vi "RandomizeTargetSequence.vi"(10 "NumRepetitions":i32, 11 "Inputs":dbl[](array[numeric])) -> (3 "Target Array":dbl[](array[numeric]))   [LabVIEW 2019]
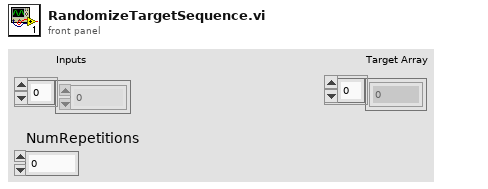
[diagram p1: front panel]
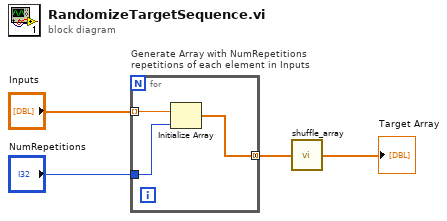
[diagram p0: block diagram]
diagram:
  n1 = for "Generate Array with NumRepetitions\nrepetitions of each element in Inputs" {
    tunnel: "Inputs" -> [w7] mode=indexing
    tunnel: "NumRepetitions" -> [w6]
    tunnel: [w5] -> w2 mode=concatenating
    n2 = Initialize Array(w7, w6) -> (w5:dbl[])
  }
  n3 = call "shuffle_array.vi"("Input Array"=w2) -> ("Shuffled Array"=→"Target Array":dbl[])
